vi "Test_WriteValue_InvalidType_Error.vi"(8 "error in (no error)":errorcluster, 11 "TestCase in":refnum<class "TestListboxItemNamesBinding.lvclass">) -> (0 "error out":errorcluster, 3 "TestCase out":refnum<class "TestListboxItemNamesBinding.lvclass">)   [LabVIEW 2017, in "TestListboxItemNamesBinding.lvclass"]
uses:
  TestListboxItemNamesBinding.lvclass
  Source/Concrete/ListboxItemNamesBinding/ListboxItemNamesBinding.lvclass/ListboxItemNamesBinding.ctl
  Source/Concrete/ListboxItemNamesBinding/ListboxItemNamesBinding.lvclass
  C:/Git/composed-transport/Source/ITransport/ITransport.lvclass
  <vilib>/Utility/error.llb/Error Cluster From Error Code.vi
  Source/ITransport/ITransport.lvclass
panel:
  out "Return Error":errorcluster
  in  "Listbox":i32(listbox)
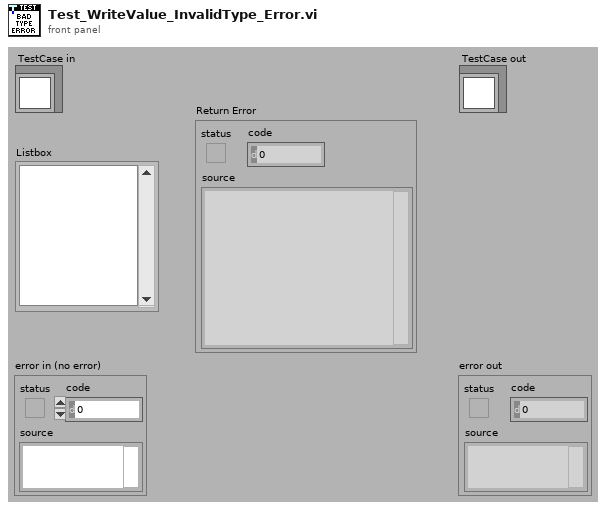
[diagram p1: front panel]
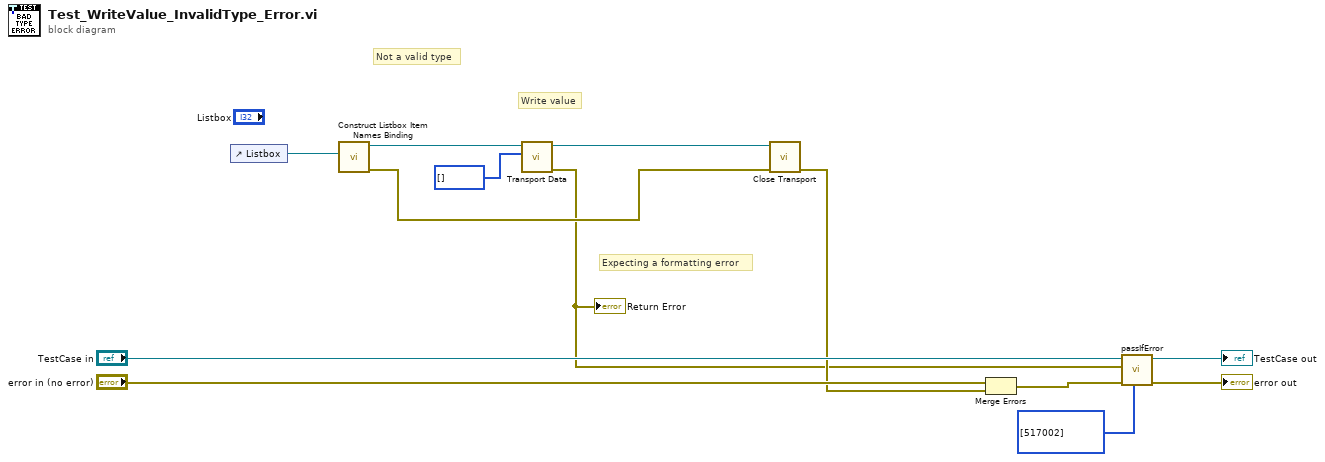
[diagram p0: block diagram]
diagram:
  # "Expecting a formatting error"
  # "Not a valid type"
  # "Write value"
  n1 = control-ref of="Listbox"() -> (w6:refnum<vi>)
  n2 = call "Construct Listbox Item Names Binding.vi"("LstBox Refnum"=w6) -> ("error out"=w3:errorcluster, "ListboxItemNamesBinding"=w9:refnum<class "ListboxItemNamesBinding.lvclass">)  [unwired: 9 in]
  n3 = call "Transport Data.vi"("Value"=i32[] [] ("Format String"), "ITransport in"=w9) -> ("error out"=w2:errorcluster, "ITransport out"=w7:refnum<class "ListboxItemNamesBinding.lvclass">)  [unwired: 8 in]
  "Return Error" <- w2
  n4 = call-dynamic "Close Transport.vi"("error in (no error)"=w3, "ITransport in"=w7) -> ("error out"=w5:errorcluster)  [unwired: 9 in]
  n5 = Merge Errors("error in (no error)", w5) -> (w8:errorcluster)
  n6 = call-dynamic "passIfError.vi"("passing error codes (default = any error code)"=i32[] [517002], "error in (no error)"=w8, "error"=w2, "TestCase in"="TestCase in") -> ("error out"=→"error out":errorcluster, "TestCase out"=→"TestCase out":refnum<class "TestListboxItemNamesBinding.lvclass">)  [unwired: 6 in]
